vi "convertChannel.vi"(1 "Channel":string) -> (0 "Channel Index":i32)   [LabVIEW 2023, in "ArbNi.lvclass"]
uses:
  ArbNi.lvclass
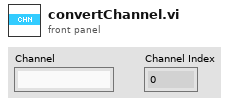
[diagram p1: front panel]
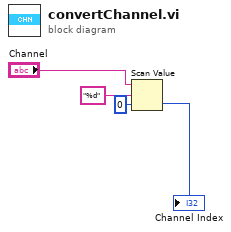
[diagram p0: block diagram]
diagram:
  n1 = Scan Value(string="Channel", format string="%d", default (0 dbl)=0) -> (value=→"Channel Index":i32)  [unwired: 1 out]
